vi "Place New Object After ID Object.vi"(7 "Named Cluster":variant, 8 "Identifying Attribute Value":string, 9 "Identifying Attribute Type":string, 10 "Element Type":string, 11 "XML String":string) -> (3 "Edited XML":string)   [LabVIEW 2019, in "EditSVG.lvclass"]
uses:
  EditSVG.lvclass
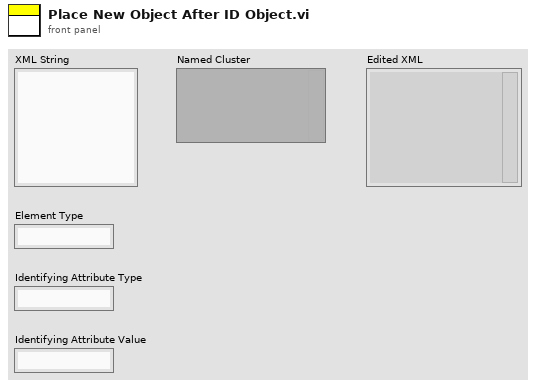
[diagram p1: front panel]
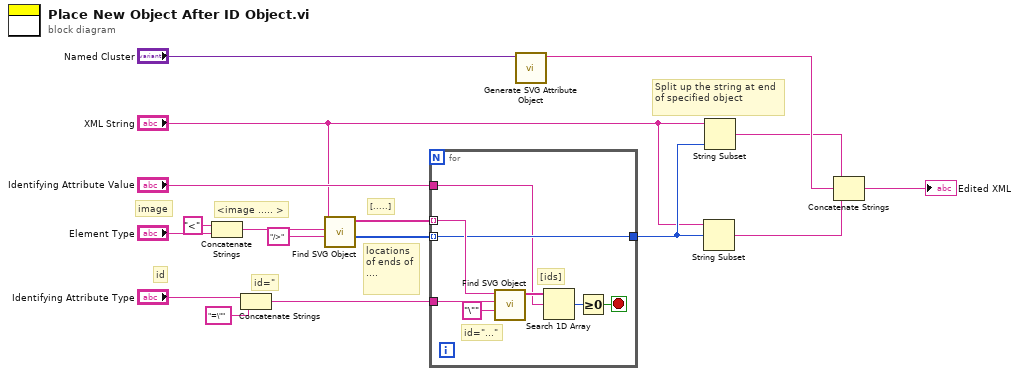
[diagram p0: block diagram]
diagram:
  # "Split up the string at end of specified object"
  # "id=\""
  # "id"
  # "locations of ends of ...."
  # "[.....]"
  # "<image ..... >"
  # "image"
  n1 = Concatenate Strings("<" ("string"), "Element Type") -> (w5:string)
  n2 = Concatenate Strings("Identifying Attribute Type", "=\"" ("string")) -> (w10:string)
  n3 = call "Find SVG Object.vi"("Ending Delimiter"="/>", "Beginning Delimiter"=w5, "XML String"="XML String") -> ("Ending Indices"=w8:i32[], "Found Values"=w16:string[])  [unwired: 6 in, 1 out]
  n4 = for {
    tunnel: w16 -> [w25] mode=indexing
    tunnel: w10 -> [w23]
    tunnel: "Identifying Attribute Value" -> [w18]
    tunnel: w8 -> [w22] mode=indexing
    tunnel: [w22] -> w4
    stop <- w19 stop-if-true
    # "id=\"...\""
    # "[ids]"
    n5 = call "Find SVG Object.vi"("Ending Delimiter"="\"", "Beginning Delimiter"=w23, "XML String"=w25) -> ("Found Values"=w21:string[])  [unwired: 6 in, 2 out]
    n6 = Search 1D Array(1D array=w21, element=w18) -> (index of element=w20:i32)  [unwired: 1 in]
    n7 = Greater Or Equal To 0?(x=w20) -> (x >= 0?=w19:bool)
  }
  n8 = call "Generate SVG Attribute Object.vi"("Named Cluster of Data"="Named Cluster") -> ("SVG Attribute Object"=w13:string)  [unwired: 9 in, 1 out]
  n9 = String Subset(string="XML String", offset (0)=w4) -> (substring=w15:string)  [unwired: 1 in]
  n10 = String Subset(string="XML String", length (rest)=w4) -> (substring=w3:string)  [unwired: 1 in]
  n11 = Concatenate Strings(w3, w13, w15) -> (→"Edited XML":string)
